vi "Creat Log File.vi"(8 "error in (no error)":errorcluster, 11 "Actor_log in":refnum<class "Actor_log.lvclass">) -> (0 "error out":errorcluster, 3 "Actor_log out":refnum<class "Actor_log.lvclass">)   [LabVIEW 2020, in "Actor_log.lvlib" / "Actor_log.lvclass"]
uses:
  Actor_log.lvclass
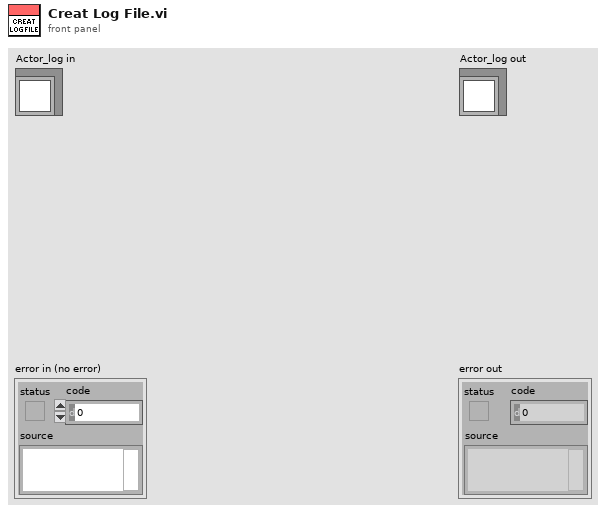
[diagram p1: front panel]
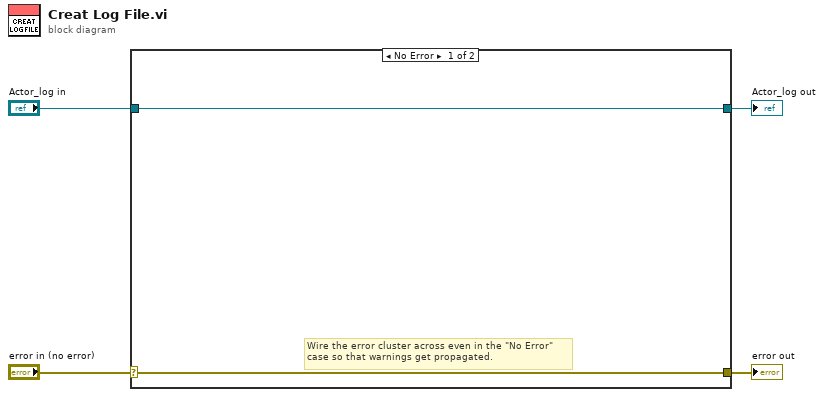
[diagram p0: block diagram]
diagram:
  n1 = case shown="No Error" "error in (no error)" {
    selector: "error in (no error)" -> [w5 w8]
    tunnel: [w5 w8] -> w3
    tunnel: [w6 w7] -> w1
    tunnel: "Actor_log in" -> [w6 w7]
    frame No Error {
      # "Wire the error cluster across even in the \"No Error\"\ncase so that warnings get propagated."
    }
    frame Error {
    }
  }
  "error out" <- w3
  "Actor_log out" <- w1
